vi "Turb参数显示.vi"() -> ()   [LabVIEW 2016, in "斯坦道多参数.lvlib"]
uses:
  <vilib>/Utility/miscctls.llb/LVPointTypeDef.ctl
panel:
  out "显示簇":T1 {"酸碱度电极零点" format="%.2f"; "电极状态标志" items=["OK", "第一点校正通过", "第二点校正通过"]; "电极型号标志" items=["NULL", "pH", "Cond", "DO", "Turb"]; "酸碱度测量值" format="%.2f"; "温度测量值" format="%.2f℃"; "酸碱度信号值" format="%.2f"; "酸碱度偏移修正值" format="%.2f"; "温度偏移修正值" format="%.2f"; "手动温度补偿值" format="%.2f"; "第1点标准值记录" format="%.2f"; "第1点信号值记录" format="%.2f"; "第1点温度值记录" format="%.2f"; "第2点标准值记录" format="%.2f"; "第2点信号值记录" format="%.2f"; "第2点温度值记录" format="%.2f"; "第一点标准值" format="%.2f"; "第二点标准值" format="%.2f"}
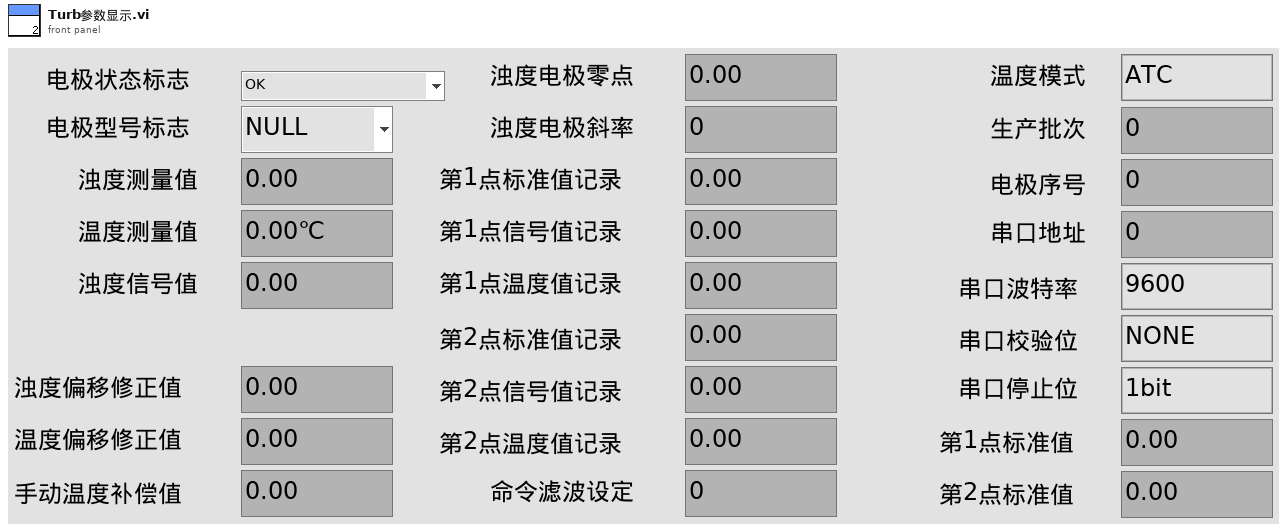
[diagram p1: front panel]
types:
  T1 = cluster{"电极状态标志":u16, "电极型号标志":u16, "酸碱度测量值":sgl, "温度测量值":sgl, "酸碱度信号值":sgl, "酸碱度偏移修正值":sgl, "温度偏移修正值":sgl, "手动温度补偿值":sgl, "酸碱度电极零点":sgl, "酸碱度电极斜率":sgl, "第1点标准值记录":sgl, "第1点信号值记录":sgl, "第1点温度值记录":sgl, "第2点标准值记录":sgl, "第2点信号值记录":sgl, "第2点温度值记录":sgl, "命令滤波设定":u16, "温度模式":enum16{"ATC", "MTC"}, "生产批次":u16, "电极序号":u16, "串口地址":u16, "串口波特率":enum16{"9600", "19200", "115200"}, "串口校验位":enum16{"NONE", "ODD", "EVEN"}, "串口停止位":enum16{"1bit", "2bit"}, "第一点标准值":sgl, "第二点标准值":sgl}
  T2 = typedef "LVPointTypeDef.ctl" = cluster{"Horizontal":i16, "Vertical":i16}
  T3 = cluster{"电极状态标志":u16, "电极型号标志":u16, "浊度测量值":sgl, "温度测量值":sgl, "浊度信号值":sgl, "浊度偏移修正值":sgl, "温度偏移修正值":sgl, "手动温度补偿值":sgl, "浊度电极零点":sgl, "浊度电极斜率":sgl, "第1点标准值记录":sgl, "第1点信号值记录":sgl, "第1点温度值记录":sgl, "第2点标准值记录":sgl, "第2点信号值记录":sgl, "第2点温度值记录":sgl, "命令滤波设定":u16, "温度模式":enum16{"ATC", "MTC"}, "生产批次":u16, "电极序号":u16, "串口地址":u16, "串口波特率":enum16{"9600", "19200", "115200"}, "串口校验位":enum16{"NONE", "ODD", "EVEN"}, "串口停止位":enum16{"1bit", "2bit"}, "第一点标准值":sgl, "第二点标准值":sgl}
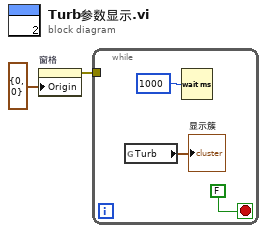
[diagram p0: block diagram]
diagram:
  n1 = property on="窗格" class="Pane"("Origin"=T2 {"Horizontal"=0, "Vertical"=0} ("原点")) -> (error out=w1:errorcluster)  [unwired: 2 in, 1 out]
  n2 = while {
    tunnel: w1 -> [_]
    stop <- FALSE stop-if-true
    n3 = global read "国弘过程全局变量.vi" "Turb"() -> (→"显示簇":T3)
    n4 = Wait (ms)(milliseconds to wait=u32 1000 ("等待时间（毫秒）")) -> ()  [unwired: 1 out]
  }
